vi "Pinch finger.vi"(6 "Multi-pinch enabled":bool, 9 "Boolean":bool, 11 "Finger Vector In":T1(array[cluster])=[{"Numeric Control"=0, "x"=0.0, "y"=0.0, "z"=0.0}, {"Numeric Control"=1, "x"=0.0, "y"=0.0, "z"=0.0}, {"Numeric Control"=2, "x"=0.0, "y"=0.0, "z"=0.0}, {"Numeric Control"=3, "x"=0.0, "y"=0.0, "z"=0.0}, {"Numeric Control"=4, "x"=0.0, "y"=0.0, "z"=0.0}]) -> (2 "Finger pinch":bool[](array[boolean]))   [LabVIEW 2014]
uses:
  <vilib>/Analysis/_algsub.llb/Vector Norm Type.ctl
  <vilib>/Analysis/_algsub.llb/Real Vector Norm.vi
  <vilib>/Analysis/NI_AALPro.lvlib
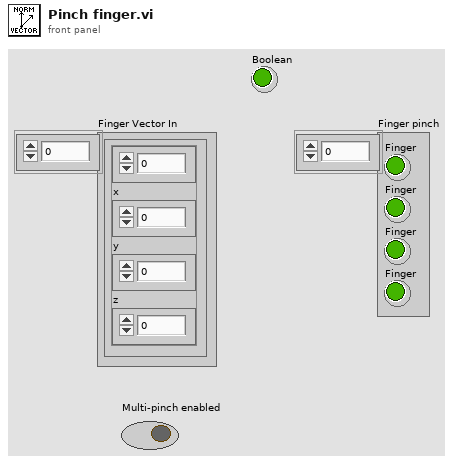
[diagram p1: front panel]
types:
  T1 = cluster{"Numeric Control":i32, "x":sgl, "y":sgl, "z":sgl}[]
  T2 = cluster{"Numeric Control":i32, "x":sgl, "y":sgl, "z":sgl}
  T3 = typedef "NI_AALPro.lvlib/Vector Norm Type.ctl" = u16
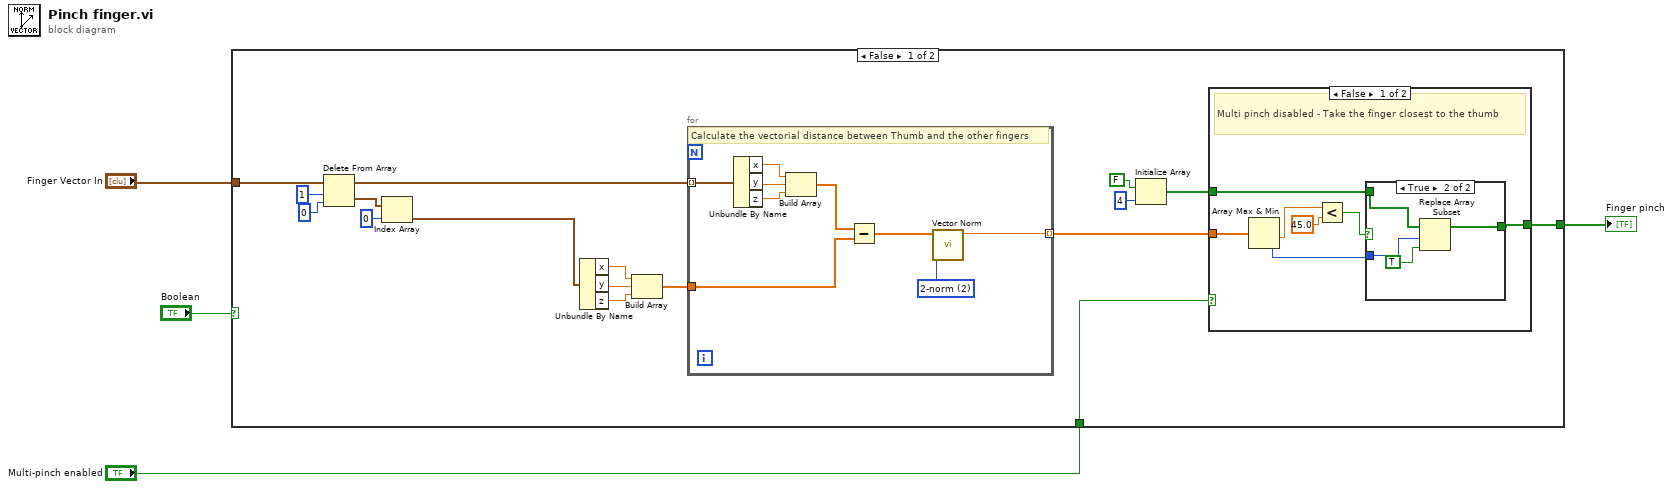
[diagram p0: block diagram]
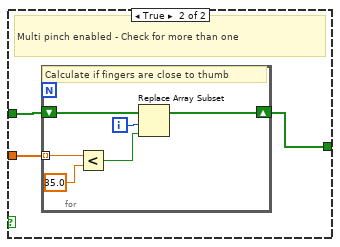
[diagram p3: hidden frame]
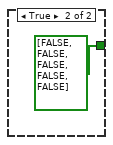
[diagram p4: hidden frame]
diagram:
  n1 = case shown="False" "Boolean" {
    tunnel: "Finger Vector In" -> [w21 _]
    tunnel: "Multi-pinch enabled" -> [w7 _]
    tunnel: [w5 bool[] [FALSE, FALSE, FALSE, FALSE, FALSE]] -> w2
    frame False {
      n2 = Delete From Array(array=w21, length=1, index=0) -> (deleted portion=w17:T1, array with subset deleted=w18:T1)
      n3 = Index Array(array=w17, index=0) -> (element=w12:T2)
      n4 = Unbundle By Name(w12) -> ("x"=w13:sgl, "y"=w14:sgl, "z"=w15:sgl)
      n5 = Build Array(w13, w14, w15) -> (w11:sgl[])
      n6 = for {
        tunnel: w18 -> [w50] mode=indexing
        tunnel: w11 -> [w45]
        tunnel: [w43] -> w10 mode=indexing
        w51 = T3 2 items=["1-norm"=1, "2-norm"=2, "Inf-norm"=3, "-Inf-norm"=4, "User Defined"=5] ("norm type")
        # "Calculate the vectorial distance between Thumb and the other fingers"
        n7 = Unbundle By Name(w50) -> ("x"=w49:sgl, "y"=w48:sgl, "z"=w47:sgl)
        n8 = Build Array(w49, w48, w47) -> (w46:sgl[])
        n9 = Subtract(x=w46, y=w45) -> (x-y=w44:sgl[])
        n10 = call-poly <vilib>:"Vector Norm.vi"("norm type"=w51, "Input Vector"=w44) -> ("norm"=w43:dbl)  [unwired: 8 in, 1 out]
      }
      n11 = Initialize Array(FALSE, 4 ("dimension size")) -> (w6:bool[])
      n12 = case shown="False" w7 {
        tunnel: w10 -> [w28 w36]
        tunnel: w6 -> [w27 w35]
        tunnel: [w26 w34] -> w5
        frame False {
          # "Multi pinch disabled - Take the finger closest to the thumb"
          n13 = Array Max & Min(array=w28) -> (min value=w24:dbl, min index (indices)=w25:i32)  [unwired: 2 out]
          n14 = Less?(x=w24, y=45.0) -> (x < y?=w22:bool)
          n15 = case shown="True" w22 {
            tunnel: w27 -> [w29 w33]
            tunnel: [w29 w31] -> w26
            tunnel: w25 -> [_ w30]
            frame False {
            }
            frame True {
              n16 = Replace Array Subset(array=w33, new element=TRUE ("new element/subarray"), index=w30) -> (w31:bool[])
            }
          }
        }
        frame True {
          # "Multi pinch enabled - Check for more than one"
          n17 = for {
            tunnel: w36 -> [w42] mode=indexing
            shift-right: [w39] -> w34
            shift-left: w35 -> [w41]
            i -> [w40]
            # "Calculate if fingers are close to thumb"
            n18 = Less?(x=w42, y=35.0) -> (x < y?=w38:bool)
            n19 = Replace Array Subset(array=w41, new element=w38, index=w40) -> (w39:bool[])
          }
        }
      }
    }
    frame True {
    }
  }
  "Finger pinch" <- w2
